vi "svl_Max-Min Level (1 Ch).vi"(8 "error in (no error)":errorcluster, 9 "processing state":T1(ring), 11 "scaled signal":waveform(dbl)={"t0"=timestamp(0 s since 1904-01-01), "dt"=0.0, "Y"=[]}) -> (0 "error out":errorcluster, 1 "max-min level":dbl format="%.2f", 2 "final min level":dbl format="%.2f", 3 "final max level":dbl format="%.2f")   [LabVIEW 2017]
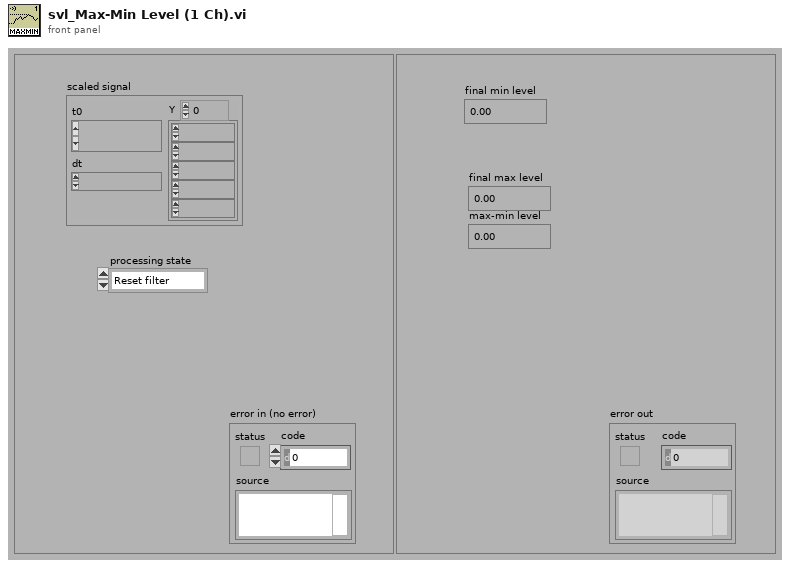
[diagram p1: front panel]
types:
  T1 = enum16{"Reset filter", "Restart averaging", "Continue processing"}
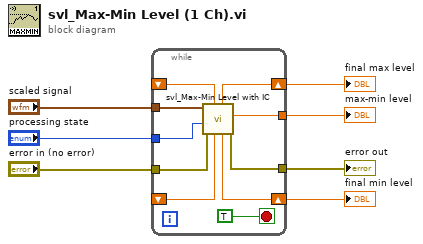
[diagram p0: block diagram]
diagram:
  n1 = while {
    tunnel: [w15] -> w4
    tunnel: "error in (no error)" -> [w16]
    tunnel: "processing state" -> [w12]
    tunnel: "scaled signal" -> [w17]
    shift-right: [w10] -> w1
    shift-left: _ -> [w11]
    shift-right: [w8] -> w2
    shift-left: _ -> [w9]
    tunnel: [w13] -> w3
    stop <- TRUE stop-if-true
    n2 = call <vilib>:"svl_Max-Min Level with IC.vi"("initial min level"=w9, "initial max level"=w11, "error in (no error)"=w16, "processing state"=w12, "scaled signal"=w17) -> ("error out"=w15:errorcluster, "max-min level"=w13:dbl, "final min level"=w8:dbl, "final max level"=w10:dbl)  [unwired: 3 in]
  }
  "final min level" <- w2
  "error out" <- w4
  "max-min level" <- w3
  "final max level" <- w1
